vi "FdxCmdMonCaptureControlCvi.vi"(7 "TriggerPosition":u32, 8 "error in":errorcluster, 9 "Strobe":u32(ring) items=["FDX_MON_STROBE_DIS", "FDX_MON_STROBE_STOP", "FDX_MON_STROBE_START"], 10 "CaptureMode":u32(ring) items=["FDX_MON_SINGLE ", "FDX_MON_CONTINUOUS", "FDX_MON_SELECTIVE", "FDX_MON_RECORDING", "FDX_MON_REROS", "FDX_MON_HMU"], 11 "InstrumentHandle_port":u32) -> (0 "error out":errorcluster, 3 "InstrumentHandle_port":u32)   [LabVIEW 2020, in "AIM664LV.lvlib"]
doc: "This function is to control the capture mode of the Monitor."
uses:
  AIM664LV.lvlib
  AFDX_LibraryAdmin/FdxGlobalDllPath.vi
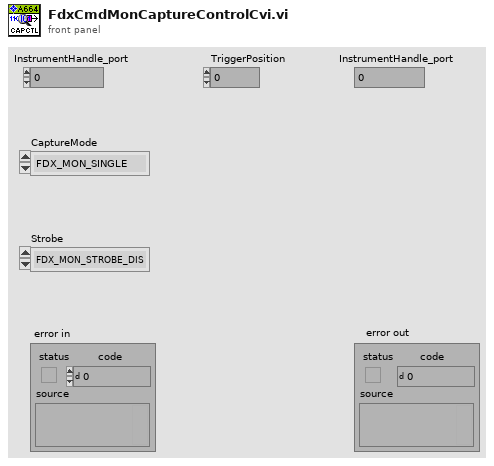
[diagram p1: front panel]
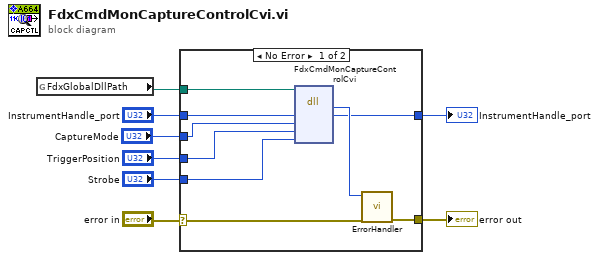
[diagram p0: block diagram]
diagram:
  n1 = global read "FdxGlobalDllPath.vi" "FdxGlobalDllPath"() -> (w6:path)
  n2 = case shown="No Error" "error in" {
    selector: "error in" -> [w16 w19]
    tunnel: [w17 w19] -> w8
    tunnel: w6 -> [w14 _]
    tunnel: "InstrumentHandle_port" -> [w13 w18]
    tunnel: [w12 w18] -> w4
    tunnel: "CaptureMode" -> [w11 _]
    tunnel: "TriggerPosition" -> [w10 _]
    tunnel: "Strobe" -> [w9 _]
    frame No Error {
      n3 = dll-call lib="aim_fdx.19.dll" fn="FdxCmdMonCaptureControlCvi"(path in=w14, "InstrumentHandle"=w13, "CaptureMode"=w11, "TriggerPosition"=w10, "Strobe"=w9) -> ("status"=w15:i32, "InstrumentHandle"=w12:u32)  [unwired: 5 in, 2 out]
      n4 = call "ErrorHandler.vi"("error in"=w16, "AIM Error"=w15) -> ("error out"=w17:errorcluster)  [unwired: 9 in]
    }
    frame Error {
    }
  }
  "error out" <- w8
  "InstrumentHandle_port" <- w4
